vi "zadanie1.vi"() -> ()   [LabVIEW 2012]
panel:
  out "Wartoœci funkcji:":dbl[][](array[numeric])
  in  "rozpocznij":bool
  in  "Podaj wartoœæ wspó³czynnika a:":dbl
  out "wykres funkcji: y = ax":cluster{i32, dbl}[](graph)
  # "Program wyznacza elementy funkcji y = ax oraz przedstawia jej wykres. \nWspó³czynnik a jest podany przez u¿ytkownika"
  # "x"
  # "y"
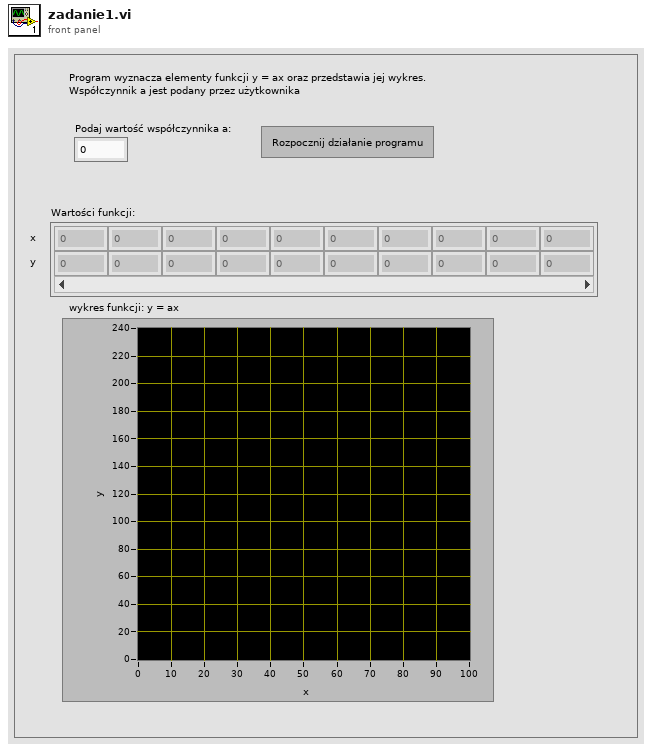
[diagram p1: front panel]
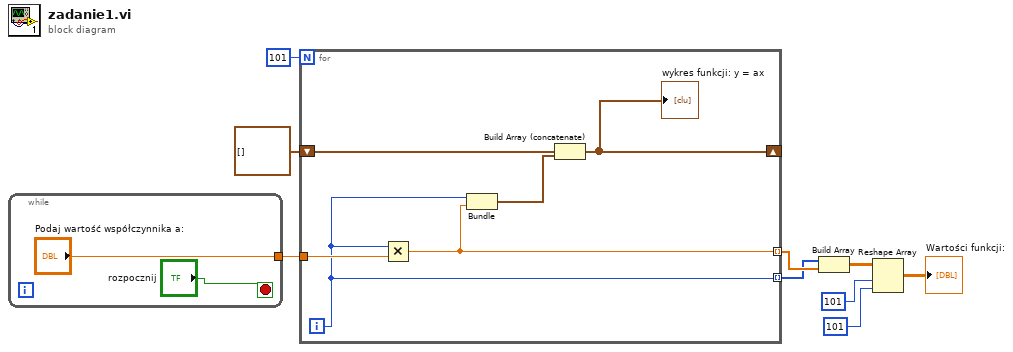
[diagram p0: block diagram]
diagram:
  n1 = while {
    tunnel: ["Podaj wartoœæ wspó³czynnika a:"] -> w8
    stop <- "rozpocznij" stop-if-true
  }
  n2 = for {
    N: 101 -> [_]
    shift-right: [w16] -> _
    shift-left: cluster{i32, i32}[] [] -> [w15]
    tunnel: w8 -> [w14]
    tunnel: [w13] -> w2 mode=indexing
    tunnel: [w12] -> w1 mode=indexing
    i -> [w12]
    n3 = Multiply(x=w12, y=w14) -> (x*y=w13:dbl)
    n4 = Bundle(w12, w13) -> (w17:cluster{i32, dbl})  [unwired: 1 in]
    n5 = Build Array (concatenate)(w15, w17) -> (w16:cluster{i32, dbl}[])
    "wykres funkcji: y = ax" <- w16
  }
  n6 = Build Array(w1, w2) -> (w5:dbl[][])
  n7 = Reshape Array(w5, 101, 101) -> (→"Wartoœci funkcji:":dbl[][])
